vi "RC_Client 3.vi"(8 "error in (no error)":errorcluster, 11 "RC Type":T1) -> (0 "error out":errorcluster)   [LabVIEW 2019, in "RemoteControl.lvclass"]
uses:
  RemoteControl.lvclass
  Typedefs/RC Com Type--enum.ctl
  f0cea44e-82f5-4e56-b32e-d2cb384a2566.vi
  db51367f-c7f3-480a-b132-7f33093295d6.vi
  d8d5aeaf-e1b8-48f3-8146-827dda1e4654.vi
  f0cea44e-82f5-4e56-b32e-d2cb384a2566.vi/34564050-70fa-4264-8484-ed8026e6cfbb.vi
  db51367f-c7f3-480a-b132-7f33093295d6.vi/7a694121-6eb5-43b4-9881-2eb32b32ed0f.vi
  d8d5aeaf-e1b8-48f3-8146-827dda1e4654.vi/7066d54e-bd41-4329-bd58-82b69b3e8ced.vi
  <vilib>/Utility/LVClass/Get LV Class Name.vi
  <vilib>/JDP Science/JSONtext/JSON text to Variant.vi
  <userlib>/_OpenG.lib/numeric/numeric.llb/Random Number Within Range - I32__ogtk.vi
  <userlib>/_OpenG.lib/error/error.llb/Filter Error Codes (Array)__ogtk.vi
  <vilib>/JDP Science/JSONtext/LVClass Serializer/JSONtext LVClass Serializer.lvclass
panel:
  in  "milliseconds to wait":u32
  out "time (1 message) (ms)":u32
  out "startup time (ms)":u32
  out "messsages/s":dbl
  in  "remote port":u16=6341
  in  "address":string
  out "Response":string
  out "Messages":i32
  in  "Stop":bool
  out "Command reponse":string
  out "Command":string
  out "meta data\n(available commands)":string
  # "CLIENT (API)"
  # "Connection info"
  # "Message Sent"
  # "Message Received"
  # "Metrics"
  # "3"
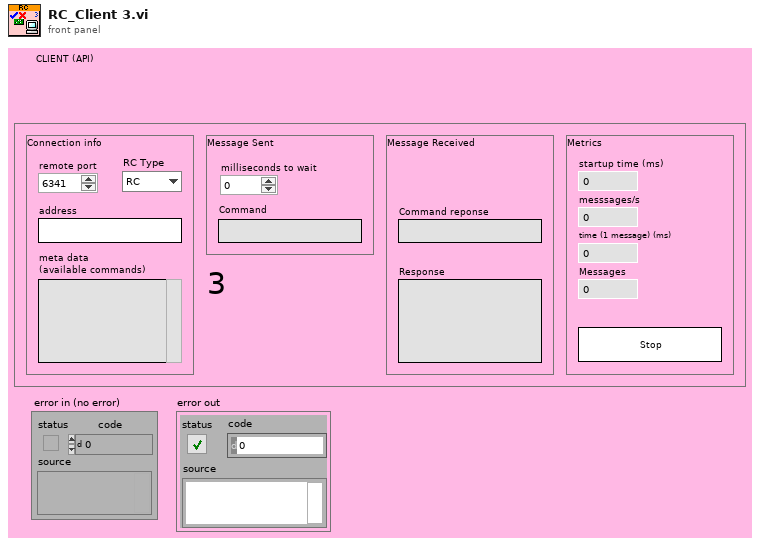
[diagram p1: front panel]
types:
  T1 = typedef "RemoteControl.lvclass/RC Com Type--enum.ctl" = enum16{"RC", "STM", "ZMQ"}
  T2 = cluster{"Command out":string, "Data out":variant, string}
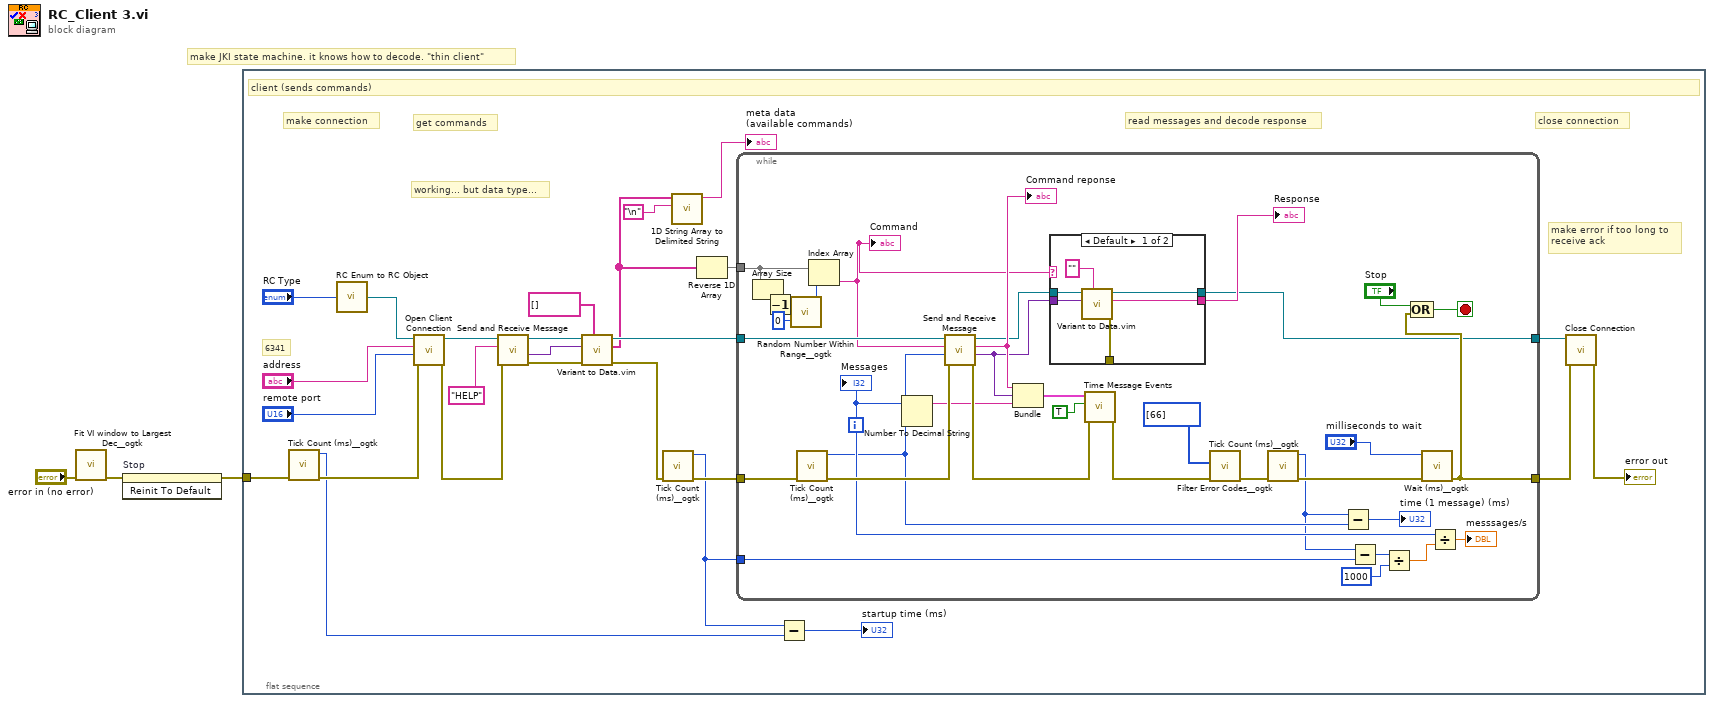
[diagram p0: block diagram]
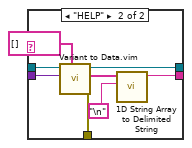
[diagram p2: hidden frame]
diagram:
  # "make JKI state machine. it knows how to decode. \"thin client\""
  n1 = call <userlib>:"Fit VI window to Largest Dec__ogtk.vi"("error in (no error)"="error in (no error)") -> ("error out"=w3:errorcluster)  [unwired: 5 in, 1 out]
  n2 = invoke on="Stop" class="Bool" method="Reinit To Default"(error in=w3) -> (error out=w2:errorcluster)  [unwired: 2 in, 2 out]
  n3 = flat-sequence {
    tunnel: w2 -> [w17]
    frame #0 {
      # "working... but data type..."
      # "close connection"
      # "read messages and decode response"
      # "get commands"
      # "make connection"
      # "6341"
      # "make error if too long to\nreceive ack"
      # "client (sends commands)"
      n4 = call <userlib>:"Tick Count (ms)__ogtk.vi"("error in (no error)"=w17) -> ("error out"=w24:errorcluster, "millisecond timer value"=w21:u32)  [unwired: 9 in]
      n5 = call "RC Enum to RC Object.vi"("RC Type"="RC Type") -> ("RemoteControl out"=w12:refnum<class "RemoteControl.lvclass">)
      n6 = call-dynamic "Open Client Connection.vi"("error in (no error)"=w24, "Port"="remote port", "address"="address", "RemoteControl in"=w12) -> ("error out"=w16:errorcluster, "RemoteControl out"=w14:refnum<class "RemoteControl.lvclass">)  [unwired: 6 in]
      n7 = call-dynamic "Send and Receive Message.vi"("error in (no error)"=w16, "Command"="HELP", "RemoteControl in"=w14) -> ("error out"=w13:errorcluster, "Data out"=w6:variant, "RemoteControl out"=w9:refnum<class "RemoteControl.lvclass">)  [unwired: 5 in, 1 out]
      n8 = call "Variant to Data.vim"("Data Type"=string[] [], "error in (no error)"=w13, "Data in"=w6, "RemoteControl in"=w9) -> ("error out"=w11:errorcluster, "Data out"=w5:string[], "RemoteControl out"=w8:refnum<class "RemoteControl.lvclass">)  [unwired: 5 in]
      n9 = call <userlib>:"Tick Count (ms)__ogtk.vi"("error in (no error)"=w11) -> ("error out"=w23:errorcluster, "millisecond timer value"=w18:u32)  [unwired: 9 in]
      n10 = call <vilib>:"1D String Array to Delimited String.vi"("delimiter"="\n", "string array"=w5) -> ("delimited string"=→"meta data\n(available commands)":string)  [unwired: 9 in]
      n11 = Reverse 1D Array(array=w5) -> (reversed array=w25:string[])
      n12 = while {
        tunnel: [w43] -> w29
        tunnel: [w32] -> w28
        tunnel: w23 -> [w58]
        tunnel: w8 -> [w62]
        tunnel: w25 -> [w47]
        tunnel: w18 -> [w37]
        i -> [w55]
        stop <- w64 stop-if-true
        n13 = Array Size(array=w47) -> (size(s)=w48:i32)
        n14 = Decrement(x=w48) -> (x-1=w46:i32)
        n15 = call-poly <userlib>:"Random Number Within Range__ogtk.vi"("High"=w46, "Low"=0) -> ("Random Number"=w50:i32)  [unwired: 3 in]
        n16 = call <userlib>:"Tick Count (ms)__ogtk.vi"("error in (no error)"=w58) -> ("error out"=w57:errorcluster, "millisecond timer value"=w44:u32)  [unwired: 9 in]
        n17 = Index Array(array=w47, index=w50) -> (element=w31:string)
        "Command" <- w31
        n18 = Number To Decimal String(number=w55) -> (decimal integer string=w30:string)  [unwired: 1 in]
        n19 = call-dynamic "Send and Receive Message.vi"("error in (no error)"=w57, "Data"=w44, "Command"=w31, "RemoteControl in"=w62) -> ("error out"=w45:errorcluster, "Data out"=w33:variant, "Command out"=w56:string, "RemoteControl out"=w34:refnum<class "RemoteControl.lvclass">)  [unwired: 4 in]
        "Command reponse" <- w56
        n20 = Bundle("Command out"=w56, "Data out"=w33, w30) -> (w54:T2)  [unwired: 1 in]
        n21 = case shown="Default" w31 {
          tunnel: [w69 w73] -> w35
          tunnel: w34 -> [w68 w77]
          tunnel: w33 -> [w67 w76]
          tunnel: [w66 w75] -> w32
          tunnel: [w65 w71] -> _
          frame Default {
            n22 = call "Variant to Data.vim"("Data Type"="", "Data in"=w67, "RemoteControl in"=w68) -> ("error out"=w65:errorcluster, "Data out"=w69:string, "RemoteControl out"=w66:refnum<class "RemoteControl.lvclass">)  [unwired: 6 in]
          }
          frame "HELP" {
            n23 = call "Variant to Data.vim"("Data Type"=string[] [], "Data in"=w76, "RemoteControl in"=w77) -> ("error out"=w71:errorcluster, "Data out"=w74:string[], "RemoteControl out"=w75:refnum<class "RemoteControl.lvclass">)  [unwired: 6 in]
            n24 = call <vilib>:"1D String Array to Delimited String.vi"("delimiter"="\n", "string array"=w74) -> ("delimited string"=w73:string)  [unwired: 9 in]
          }
        }
        "Response" <- w35
        n25 = call "Time Message Events.vi"("error in (no error)"=w45, "Debug Mode"=TRUE, "Message in"=w54) -> ("error out"=w36:errorcluster)  [unwired: 6 in, 2 out]
        n26 = call-poly <userlib>:"Filter Error Codes__ogtk.vi"("Error In"=w36, "Error Codes to Filter"=i32[] [66]) -> ("Error Out"=w61:errorcluster)  [unwired: 7 in, 2 out]
        n27 = call <userlib>:"Tick Count (ms)__ogtk.vi"("error in (no error)"=w61) -> ("error out"=w52:errorcluster, "millisecond timer value"=w39:u32)  [unwired: 9 in]
        n28 = Subtract(x=w39, y=w44) -> (x-y=→"time (1 message) (ms)":u32)
        n29 = Subtract(x=w39, y=w37) -> (x-y=w38:u32)
        n30 = Divide(x=w38, y=u32 1000) -> (x/y=w60:dbl)
        n31 = call <userlib>:"Wait (ms)__ogtk.vi"("error in (no error)"=w52, "milliseconds to wait"="milliseconds to wait") -> ("error out"=w43:errorcluster)  [unwired: 8 in, 1 out]
        n32 = Compound Arithmetic op=OR("Stop", w43) -> (w64:bool)
        n33 = Divide(x=w55, y=w60) -> (x/y=→"messsages/s":dbl)
        "Messages" <- w55
      }
      n34 = Subtract(x=w18, y=w21) -> (x-y=→"startup time (ms)":u32)
      n35 = call-dynamic "Close Connection.vi"("error in (no error)"=w29, "RemoteControl in"=w28) -> ("error out"=→"error out":errorcluster)  [unwired: 8 in, 1 out]
    }
  }
